vi "ChangeRefreshGraphicsState.vi"(8 "error in (no error)":errorcluster, 9 "refreshing?":bool, 10 "button ref":refnum<vi>, 11 "animatedDecoration ref":refnum<vi>) -> (0 "error out":errorcluster)   [LabVIEW 2021]
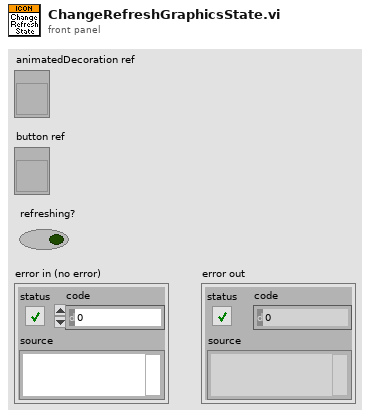
[diagram p1: front panel]
types:
  T1 = enum8{"Enabled", "Disabled", "Disabled and Grayed Out"}
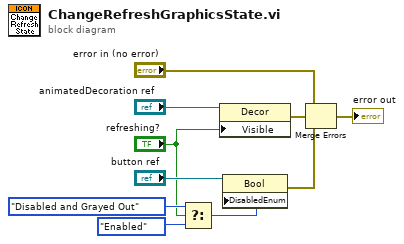
[diagram p0: block diagram]
diagram:
  n1 = Select(t=T1."Disabled and Grayed Out" ("Disabled"), s="refreshing?", f=T1."Enabled" ("Disabled")) -> (s? t:f=w6:T1)
  n2 = property class="Decor"(reference="animatedDecoration ref", "Visible"="refreshing?") -> (error out=w3:errorcluster)  [unwired: 1 in, 1 out]
  n3 = property class="Bool"(reference="button ref", "DisabledEnum"=w6) -> (error out=w4:errorcluster)  [unwired: 1 in, 1 out]
  n4 = Merge Errors("error in (no error)", w3, w4) -> (→"error out":errorcluster)
